vi "dtrsm - Solve Linear Eqs (Triangle, multiple) (DBL).vi"(4 "diagonal":T3 items=["Non-unit", "Unit"], 5 "side":T1=1 items=["Left"=1, "Right"=0], 6 "alpha":dbl=1.0, 7 "operation A":T5 items=["Direct", "Conjugated & Transposed", "Transposed"], 8 "matrix A type":T4=3 items=["Lower Triangular"=2, "Upper Triangular"=3], 10 "x":T2, 11 "A":T2) -> (0 "error":i32, 3 "dtrsm":T2)   [LabVIEW 2017, in "NI_AALBLAS.lvlib"]
doc: "Solves either op(A)*<B>trsm</B> = <B>alpha</B>*<B>x</B> or <B>trsm</B>*op(A) = <B>alpha</B>*<B>x</B> for <B>trsm</B>."
uses:
  NI_AALBLAS.lvlib
  RealMatrix.ctl
  LV_Transpose.ctl
  LV_UpLo.ctl
  LV_Diag.ctl
  LV_Side.ctl
  Fucntion.ctl
  Order.ctl
  BLAS3 Utility(DBL).vi
  NI_Matrix.lvlib
panel:
  # "-1"
  # "-1"
  # "dtrsm=alpha*op(A)  *X / dtrsm=alpha*X*op(A)"
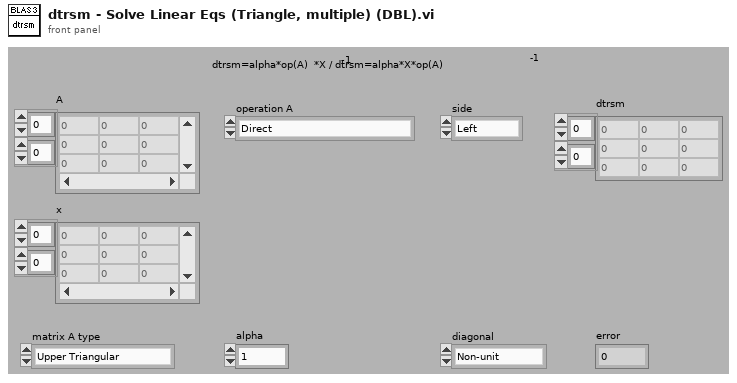
[diagram p1: front panel]
types:
  T1 = typedef "NI_AALBLAS.lvlib/LV_Side.ctl" = i32
  T2 = typedef "NI_Matrix.lvlib/RealMatrix.ctl" = dbl[][]
  T3 = typedef "NI_AALBLAS.lvlib/LV_Diag.ctl" = i32
  T4 = typedef "NI_AALBLAS.lvlib/LV_UpLo.ctl" = i32
  T5 = typedef "NI_AALBLAS.lvlib/LV_Transpose.ctl" = i32
  T6 = typedef "NI_AALBLAS.lvlib/Order.ctl" = i32
  T7 = typedef "NI_AALBLAS.lvlib/Fucntion.ctl" = u16
  T8 = typedef "NI_AALBLAS.lvlib/Diag.ctl" = i32
  T9 = typedef "NI_AALBLAS.lvlib/Operation_Transpose.ctl" = i32
  T10 = typedef "NI_AALBLAS.lvlib/UpLo.ctl" = i32
  T11 = typedef "NI_AALBLAS.lvlib/Side.ctl" = i32
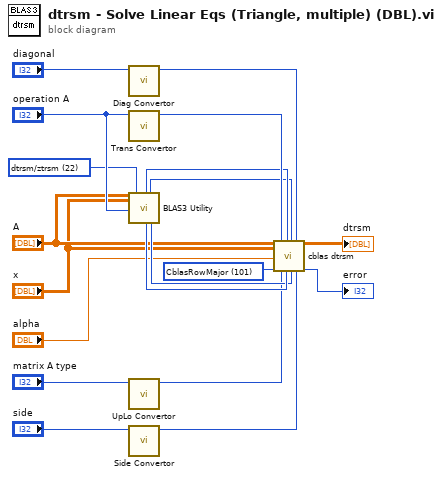
[diagram p0: block diagram]
diagram:
  w1 = T6 101 items=["CblasRowMajor"=101, "CblasColMajor"=102] ("order")
  w4 = T7 22 items=["ddot/zdotu/zdotc", "daxpy/zaxpy", "dnrm2/dznrm2", "dasum/dzasum", "dcopy/zcopy", "dswap/zswap", "drotm", "drot/zdrot", "idamax/izamax", "idamin/izamin", "dgemv/zgemv", "dsymv/zhemv", "dtrmv/ztrmv", "dsyr/zher", "dsyr2/zher2", "dger/zgeru/zgerc", "dtrsv/ztrsv", "dgemm/zgemm", "dsymm/zsymm/zhemm", "dtrmm/ztrmm", "dsyrk/zsyrk/zherk", "dsyr2k/zsyr2k/zher2k", "dtrsm/ztrsm"] ("function")
  n1 = call "Diag Convertor.vi"("diagonal"="diagonal") -> ("diag"=w12:T8)  [unwired: 10 out]
  n2 = call "Trans Convertor.vi"("operation"="operation A") -> ("trans"=w11:T9)  [unwired: 10 out]
  n3 = call-poly "BLAS3 Utility.vi"("A"="A", "B/X"="x", "operation A"="operation A", "function"=w4) -> ("lda"=w3:i32, "m"=w18:i32, "ldb/ldx"=w2:i32, "n"=w17:i32)  [unwired: 2 in, 10 out]
  n4 = call "UpLo Convertor.vi"("triangle matrix type"="matrix A type") -> ("uplo"=w15:T10)  [unwired: 10 out]
  n5 = call "Side Convertor.vi"("LV side"="side") -> ("side"=w9:T11)  [unwired: 10 out]
  n6 = call "cblas dtrsm.vi"("A"="A", "x"="x", "alpha"="alpha", "order"=w1, "transA"=w11, "uplo"=w15, "lda"=w3, "m"=w18, "ldx"=w2, "n"=w17, "diag"=w12, "side"=w9) -> ("dtrsm"=→"dtrsm":T2, "error"=→"error":i32)  [unwired: 6 out]
